vi "XIPIN_Utility_Buffer_2_1.vi"   [LabVIEW 2017]
doc: "Utility ip for instantiating various Buffers, such as BUFG, differential IO Buffers etc.\n------------------------------------\n<b>Need License</b> : No"
uses:
  <vilib>/rvi/XilinxIP/XIPIN_XNode/niFpgaXIPIN.xnode
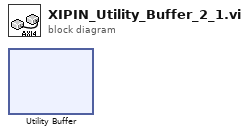
[diagram p0: block diagram]
diagram:
  n1 = xnode ("Utility Buffer")() -> ()
